vi "Limit Servings.vi"(11 "servings":i32) -> (3 "coerced":i32)   [LabVIEW 2019, in "Pet Feeder.lvlib"]
uses:
  Pet Feeder.lvlib
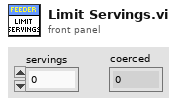
[diagram p1: front panel]
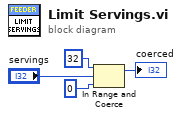
[diagram p0: block diagram]
diagram:
  n1 = In Range and Coerce(upper limit=32, x="servings", lower limit=0) -> (coerced(x)=→"coerced":i32)  [unwired: 1 out]
